vi "Calibration Offset.vi"(7 "Relative Position":T1={"Direction"=enum."Negative", "D"=100.0} {"D" min=1.0 step=1.0}, 8 "error in (no error)":errorcluster, 9 "Calibraion Position In":cluster{"X":dbl, "Y":dbl}[](array[cluster]), 10 "Real Position":cluster{"X":dbl, "Y":dbl}[](array[cluster])) -> (0 "error out":errorcluster, 1 "Calibraion Position Out":cluster{"X":dbl, "Y":dbl}[](array[cluster]))   [LabVIEW 2019]
uses:
  <vilib>/vision/NI_Vision_Development_Module.lvlib
panel:
  in  "Relative Position":T2
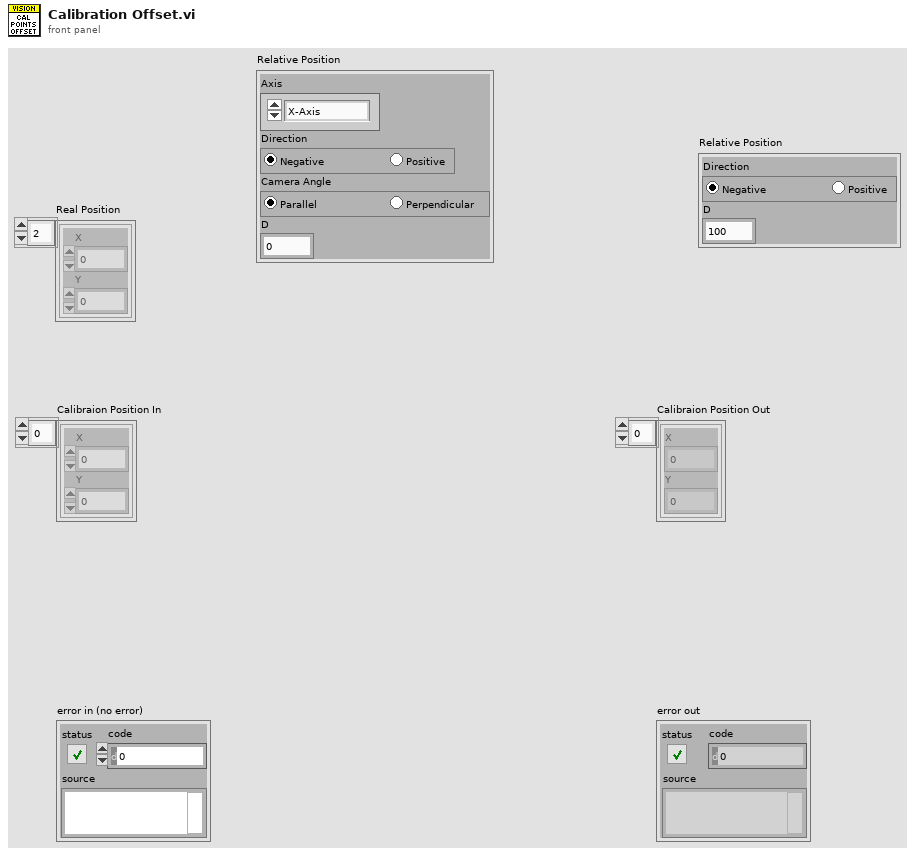
[diagram p1: front panel]
types:
  T1 = cluster{"Direction":enum32{"Negative", "Positive"}, "D":dbl}
  T2 = cluster{"Axis":enum16{"X-Axis", "Y-Axis"}, "Direction":enum32{"Negative", "Positive"}, "Camera Angle":enum32{"Parallel", "Perpendicular"}, "D":dbl}
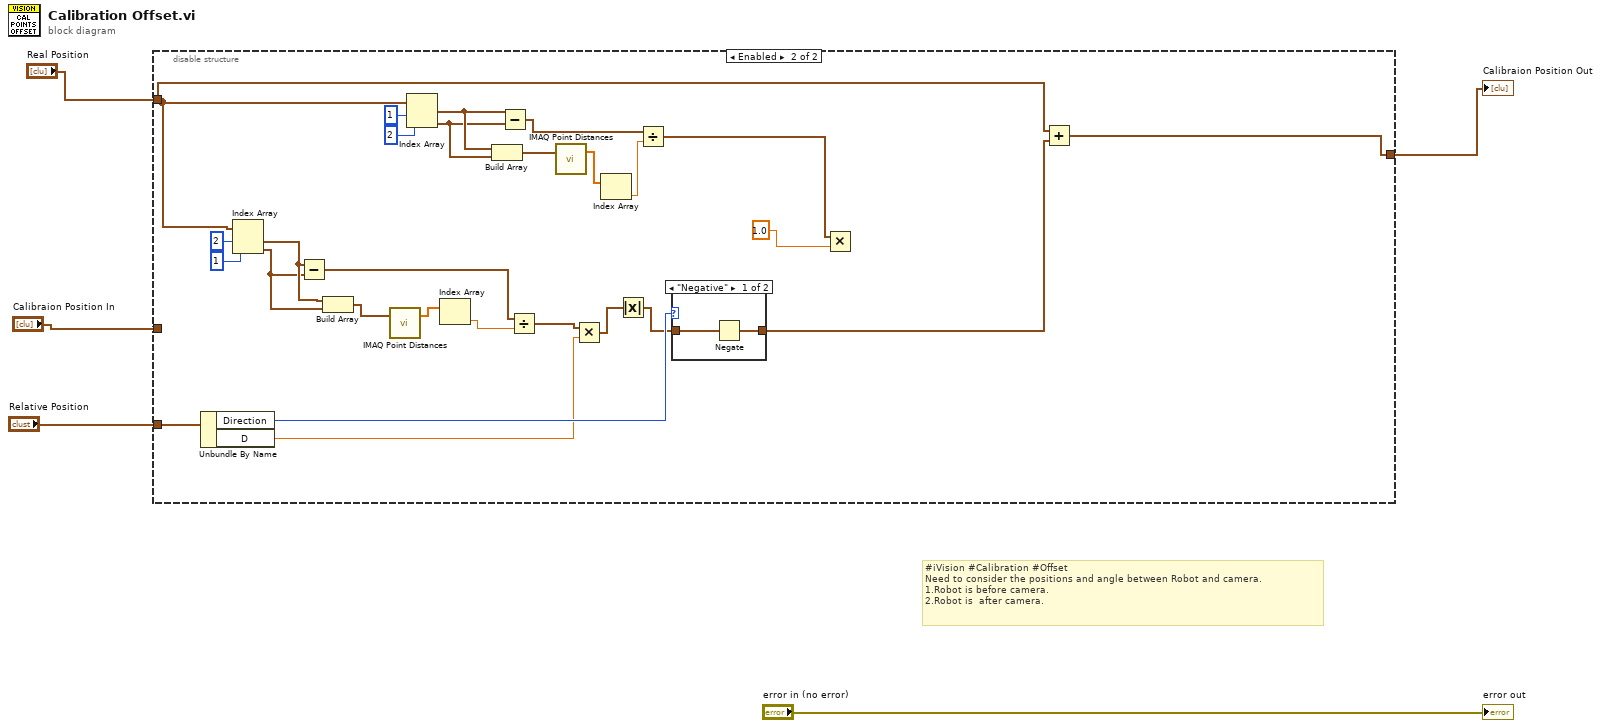
[diagram p0: block diagram]
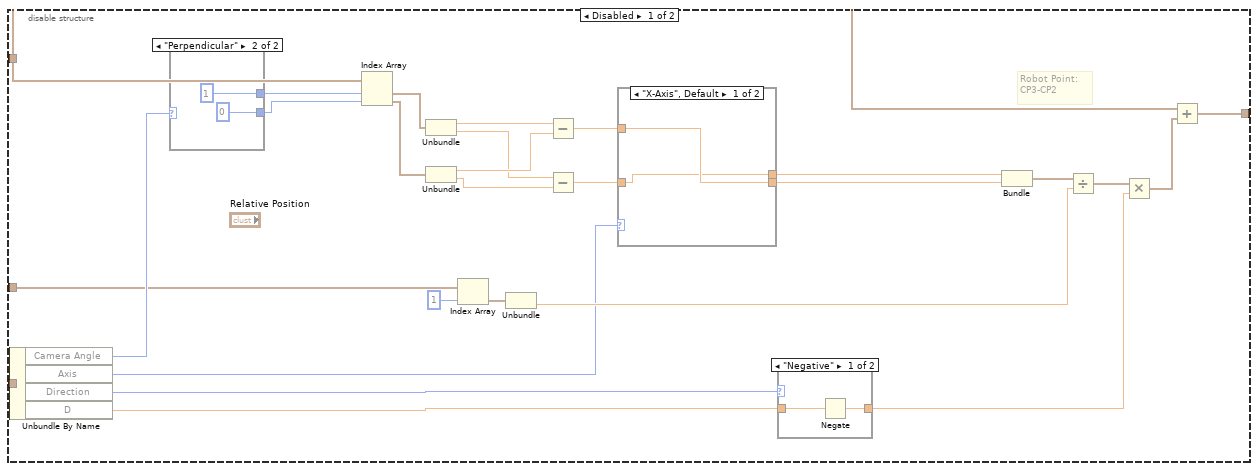
[diagram p2: hidden frame]
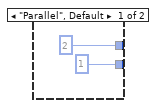
[diagram p3: hidden frame]
diagram:
  # "#iVision #Calibration #Offset\nNeed to consider the positions and angle between Robot and camera.\n1.Robot is before camera.\n2.Robot is  after camera."
  n1 = disable-structure shown="Enabled" {
    disable-tunnel: "Real Position" -> [w29 w56]
    disable-tunnel: [w19 w59] -> w4
    disable-tunnel: "Relative Position" -> [w18 w62]
    disable-tunnel: "Calibraion Position In" -> [w6 _]
    frame Disabled {
      # "Robot Point:\nCP3-CP2"
      n2 = Unbundle By Name(w18) -> ("Camera Angle"=w9:enum32{"Parallel", "Perpendicular"}, "Axis"=w14:enum16{"X-Axis", "Y-Axis"}, "Direction"=w17:enum32{"Negative", "Positive"}, "D"=w16:dbl)
      n3 = case shown="\"Perpendicular\"" w9 {
        tunnel: [2 ("index") 1 ("index")] -> w8
        tunnel: [1 ("index") 0 ("index")] -> w7
        frame "Parallel", Default {
        }
        frame "Perpendicular" {
        }
      }
      n4 = Index Array(array=w29, index #1=w8, index #2=w7) -> (element #1=w32:cluster{"X":dbl, "Y":dbl}, element #2=w31:cluster{"X":dbl, "Y":dbl})
      n5 = Unbundle(w32) -> ("X"=w26:dbl, "Y"=w27:dbl)
      n6 = Unbundle(w31) -> ("X"=w30:dbl, "Y"=w28:dbl)
      n7 = Index Array(array=w6, index=1) -> (element=w21:cluster{"X":dbl, "Y":dbl})
      n8 = Unbundle(w21) -> ("Y"=w15:dbl)  [unwired: 1 out]
      n9 = Subtract(x=w26, y=w30) -> (x-y=w13:dbl)
      n10 = Subtract(x=w27, y=w28) -> (x-y=w12:dbl)
      n11 = case shown="\"X-Axis\", Default" w14 {
        tunnel: w13 -> [w38 w39]
        tunnel: w12 -> [w37 w40]
        tunnel: [w38 w40] -> w11
        tunnel: [w37 w39] -> w10
        frame "X-Axis", Default {
        }
        frame "Y-Axis" {
        }
      }
      n12 = case shown="\"Negative\"" w17 {
        tunnel: [w42 w43] -> w25
        tunnel: w16 -> [w41 w43]
        frame "Negative" {
          n13 = Negate(x=w41) -> (-x=w42:dbl)
        }
        frame "Positive", Default {
        }
      }
      n14 = Bundle(w10, w11) -> (w24:cluster{dbl, dbl})  [unwired: 1 in]
      n15 = Divide(x=w24, y=w15) -> (x/y=w20:cluster{dbl, dbl})
      n16 = Multiply(x=w20, y=w25) -> (x*y=w23:cluster{dbl, dbl})
      n17 = Add(x=w29, y=w23) -> (x+y=w19:cluster{dbl, dbl}[])
    }
    frame Enabled {
      n18 = Unbundle By Name(w62) -> ("Direction"=w61:enum32{"Negative", "Positive"}, "D"=w54:dbl)
      n19 = Index Array(array=w56, index #1=2 ("index"), index #2=1 ("index")) -> (element #1=w48:cluster{"X":dbl, "Y":dbl}, element #2=w47:cluster{"X":dbl, "Y":dbl})
      n20 = Subtract(x=w48, y=w47) -> (x-y=w55:cluster{"X":dbl, "Y":dbl})
      n21 = Build Array(w48, w47) -> (w46:cluster{"X":dbl, "Y":dbl}[])
      n22 = call "IMAQ Point Distances"("Points"=w46) -> ("Distances"=w45:sgl[])  [unwired: 4 in, 1 out]
      n23 = Index Array(array=w56, index #1=1 ("index"), index #2=2 ("index")) -> (element #1=w68:cluster{"X":dbl, "Y":dbl}, element #2=w67:cluster{"X":dbl, "Y":dbl})
      n24 = Index Array(array=w45) -> (element=w44:sgl)  [unwired: 1 in]
      n25 = Build Array(w68, w67) -> (w66:cluster{"X":dbl, "Y":dbl}[])
      n26 = Subtract(x=w68, y=w67) -> (x-y=w65:cluster{"X":dbl, "Y":dbl})
      n27 = Divide(x=w55, y=w44) -> (x/y=w53:cluster{"X":dbl, "Y":dbl})
      n28 = call "IMAQ Point Distances"("Points"=w66) -> ("Distances"=w64:sgl[])  [unwired: 4 in, 1 out]
      n29 = Multiply(x=w53, y=w54) -> (x*y=w52:cluster{"X":dbl, "Y":dbl})
      n30 = Index Array(array=w64) -> (element=w63:sgl)  [unwired: 1 in]
      n31 = Absolute Value(x=w52) -> (abs(x)=w50:cluster{"X":dbl, "Y":dbl})
      n32 = Divide(x=w65, y=w63) -> (x/y=w60:cluster{"X":dbl, "Y":dbl})
      n33 = case shown="\"Negative\"" w61 {
        tunnel: [w72 w73] -> w49
        tunnel: w50 -> [w71 w73]
        frame "Negative" {
          n34 = Negate(x=w71) -> (-x=w72:cluster{"X":dbl, "Y":dbl})
        }
        frame "Positive", Default {
        }
      }
      n35 = Multiply(x=w60, y=1.0 ("D")) -> ()  [unwired: 1 out]
      n36 = Add(x=w56, y=w49) -> (x+y=w59:cluster{"X":dbl, "Y":dbl}[])
    }
  }
  "Calibraion Position Out" <- w4
  "error out" <- "error in (no error)"
